vi "gentec-M-Link.Set Zero.vi"(0 "VISA resource (In)":refnum<visa-resource-name>, 5 "error in (no error)":errorcluster) -> (11 "Data Read":string, 13 "Read Timeout":bool, 14 "VISA resource (Out)":refnum<visa-resource-name>, 15 "Range":T1 items=["1f", "3f", "10f", "30f", "100f", "300f", "1p", "3p", "10p", "30p", "100p", "300p", "1n", "3n", "10n", "30n", "100n", "300n", "1u", "3u", "10u", "30u", "100u", "300u", "1m", "3m", "10m", "30m", "100m", "300m", "1", "3", "10", "30", "100", "300", "1K", "3K", "10K", "30K", "100K", "300K", "1M", "3M", "10M", "30M", "100M", "300M"], 16 "Offset [V]":dbl, 17 "ADC counts":u32, 18 "Success":bool, 19 "error out":errorcluster)   [LabVIEW 2014, in "gentec-M-Link - Driver.lvlib"]
doc: "Data to write: zro\n\nCommand only. Sets the DC offset of the signal to the desired value. Reply m,n,o where m, n and o are numbers: m is Range index, n is Offset DAC code, and o is ADC counts."
uses:
  gentec-M-Link - Driver.lvlib
  Type Defs/gentec-M-Link.Range.ctl
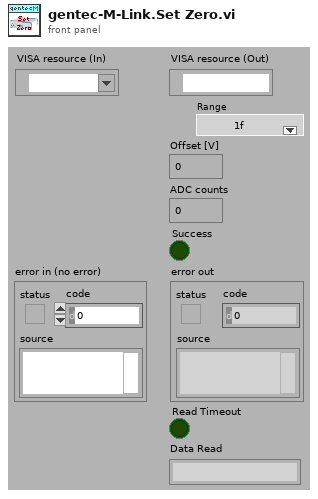
[diagram p1: front panel]
types:
  T1 = typedef "gentec-M-Link - Driver.lvlib/gentec-M-Link.Range.ctl" = u16
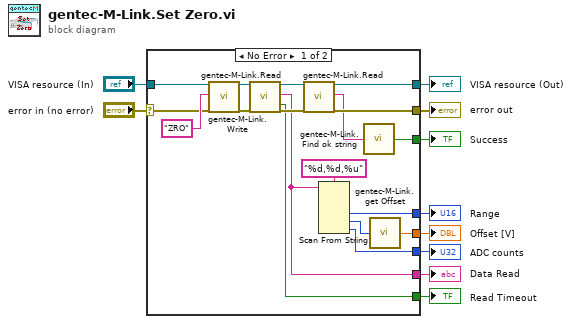
[diagram p0: block diagram]
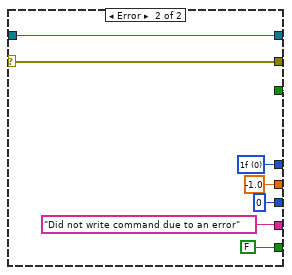
[diagram p2: hidden frame]
diagram:
  n1 = case shown="No Error" "error in (no error)" {
    selector: "error in (no error)" -> [w27 w36]
    tunnel: [w19 w36] -> w10
    tunnel: "VISA resource (In)" -> [w26 w35]
    tunnel: [w21 w35] -> w7
    tunnel: [w17 FALSE ("Found")] -> w6
    tunnel: [w16 w33] -> w5
    tunnel: [w13 -1.0] -> w4
    tunnel: [w15 u32 0] -> w3
    tunnel: [w12 FALSE ("Read Timeout")] -> w2
    tunnel: [w11 "Did not write command due to an error" ("Data Read")] -> w1
    frame No Error {
      n2 = call "gentec-M-Link.Write.vi"("VISA resource (In)"=w26, "Data To Write"="ZRO" ("format string"), "error in (no error)"=w27) -> ("VISA resource (Out)"=w24:refnum<visa-resource-name>, "error out"=w23:errorcluster)  [unwired: 14 in, 1 out]
      n3 = call "gentec-M-Link.Read.vi"("VISA resource (In)"=w24, "error in (no error)"=w23) -> ("VISA resource (Out)"=w22:refnum<visa-resource-name>, "Data Read"=w11:string, "Read Timeout"=w12:bool, "error out"=w20:errorcluster)  [unwired: 13 in, 1 out]
      n4 = call "gentec-M-Link.Read.vi"("VISA resource (In)"=w22, "error in (no error)"=w20) -> ("VISA resource (Out)"=w21:refnum<visa-resource-name>, "Data Read"=w18:string, "error out"=w19:errorcluster)  [unwired: 13 in, 2 out]
      n5 = Scan From String(format string="%d,%d,%u", input string=w11) -> (output 1=w16:i32, output 2=w14:i32, output 3=w15:u32)  [unwired: 5 in, 3 out]
      n6 = call "gentec-M-Link.Find ok string.vi"("string"=w18) -> ("Found"=w17:bool)
      n7 = call "gentec-M-Link.get Offset.vi"("Offset DAC Code"=w14) -> ("Offset [V]"=w13:dbl)
    }
    frame Error {
      w33 = T1 0 items=["1f", "3f", "10f", "30f", "100f", "300f", "1p", "3p", "10p", "30p", "100p", "300p", "1n", "3n", "10n", "30n", "100n", "300n", "1u", "3u", "10u", "30u", "100u", "300u", "1m", "3m", "10m", "30m", "100m", "300m", "1", "3", "10", "30", "100", "300", "1K", "3K", "10K", "30K", "100K", "300K", "1M", "3M", "10M", "30M", "100M", "300M", "Auto"]
    }
  }
  "error out" <- w10
  "VISA resource (Out)" <- w7
  "Success" <- w6
  "Range" <- w5
  "Offset [V]" <- w4
  "ADC counts" <- w3
  "Read Timeout" <- w2
  "Data Read" <- w1
